vi "v2 Elevador.vi"() -> ()   [LabVIEW 2018]
panel:
  in  "Alarma":bool
  in  "NIVEL 2 2":bool
  in  "NIVEL 2 1":bool
  in  "NIVEL1 2":bool
  in  "NIVEL 1 1":bool
  in  "PLANTA BAJA 2":bool
  in  "PLANTA BAJA 1":bool
  in  "A piso 2":bool
  in  "A piso 1":bool
  in  "A planta Baja":bool
  out "Puertas Abiertas":bool
  out "Nivel actual":string
  in  "Piso 2":bool
  in  "Piso 1":bool
  in  "Planta baja":bool
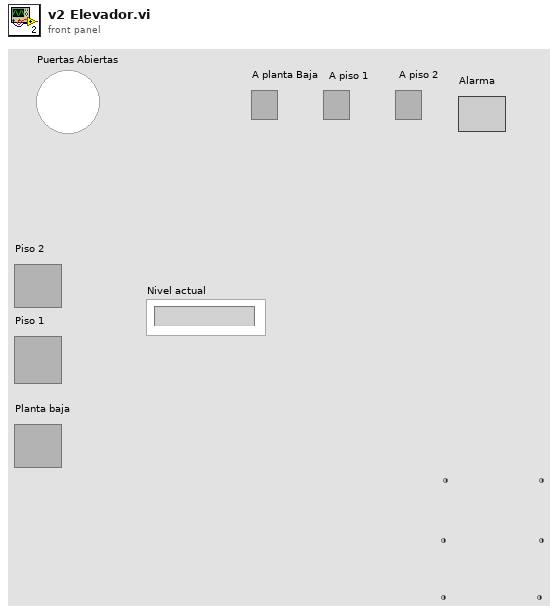
[diagram p1: front panel]
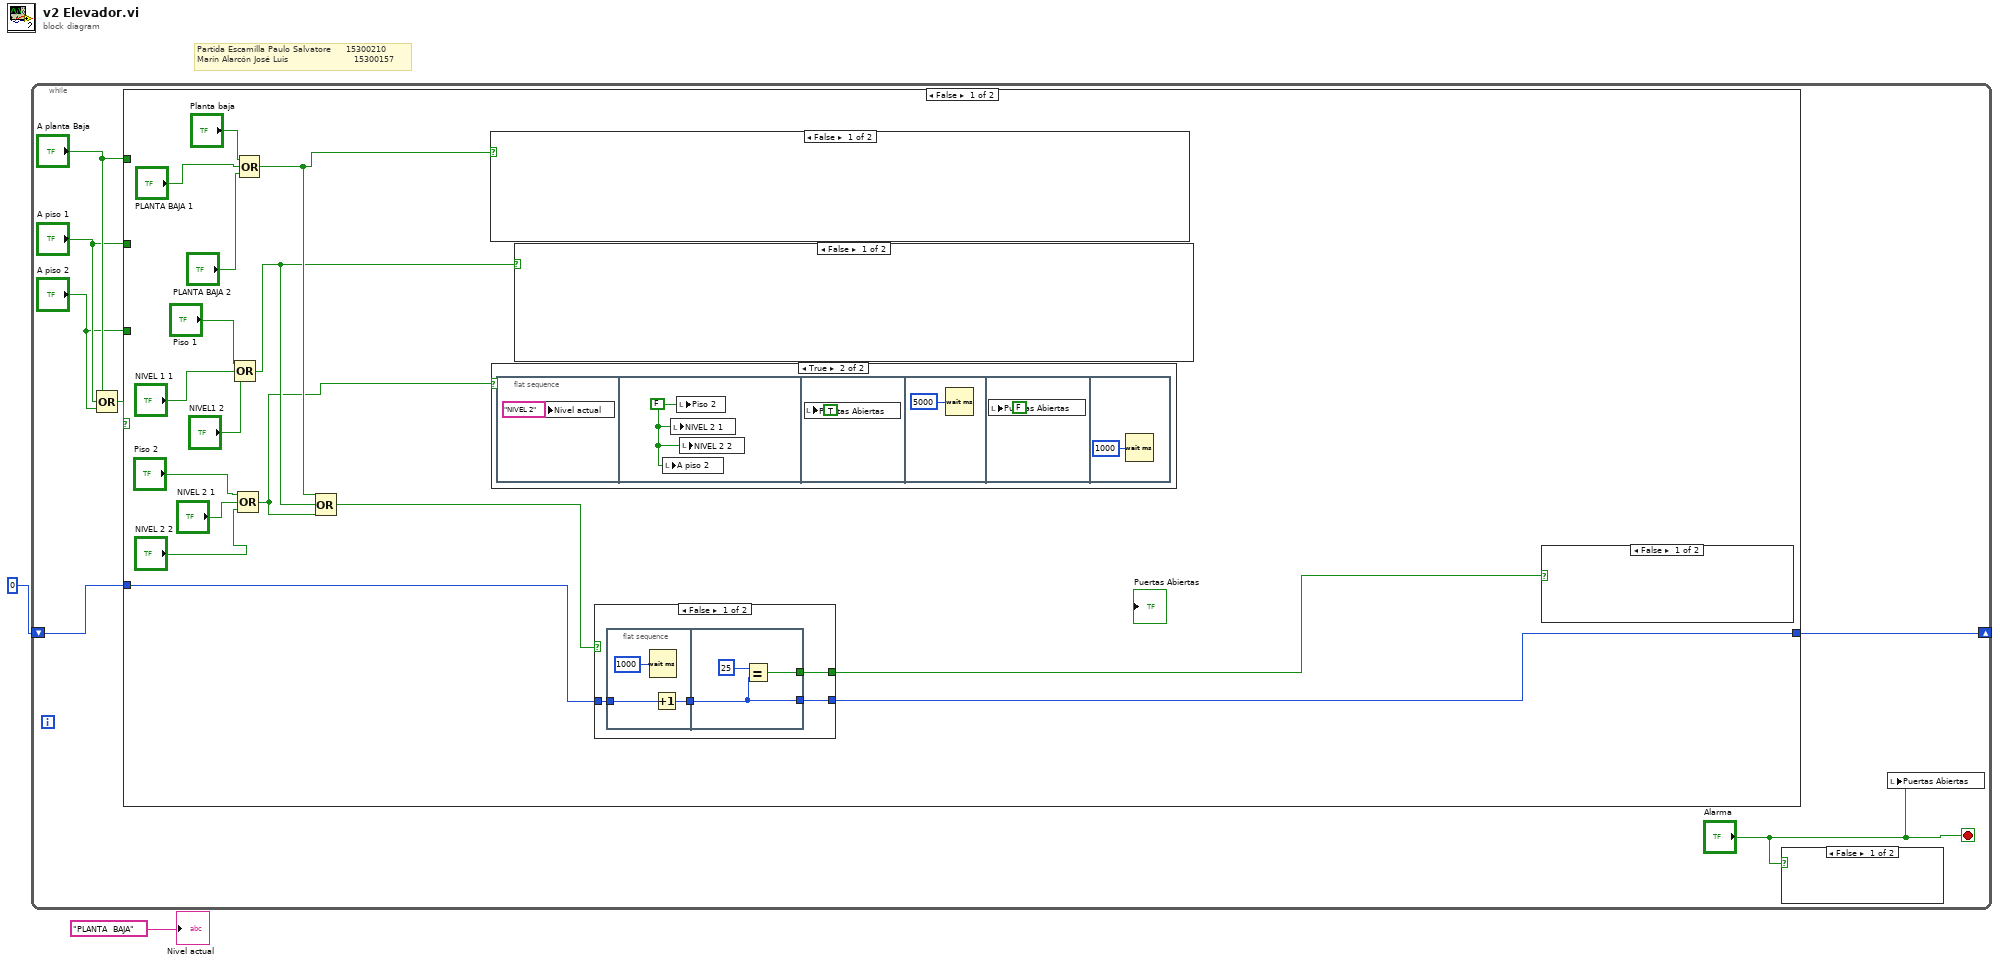
[diagram p0: block diagram]
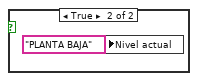
[diagram p2: hidden frame]
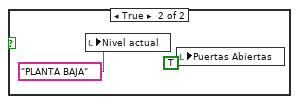
[diagram p3: hidden frame]
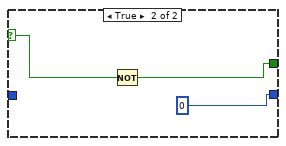
[diagram p4: hidden frame]
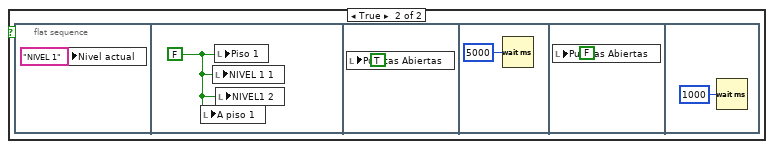
[diagram p6: hidden frame]
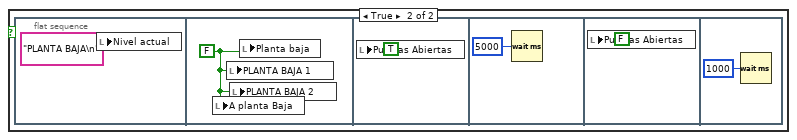
[diagram p7: hidden frame]
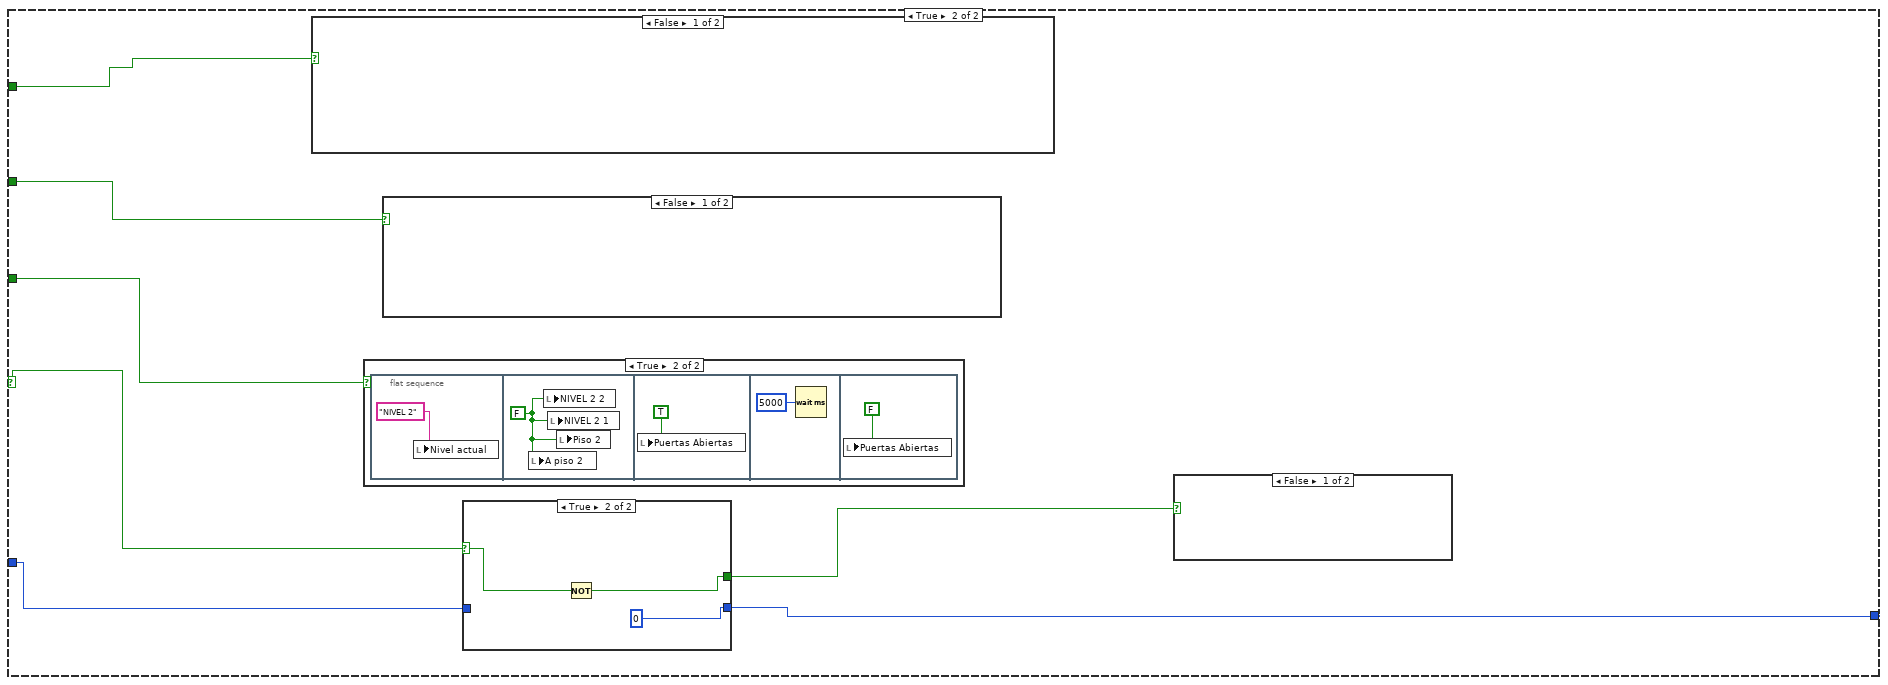
[diagram p8: hidden frame]
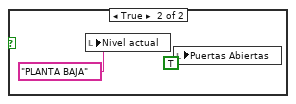
[diagram p9: hidden frame]
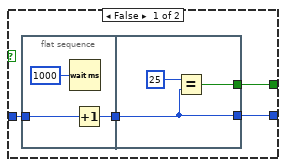
[diagram p10: hidden frame]
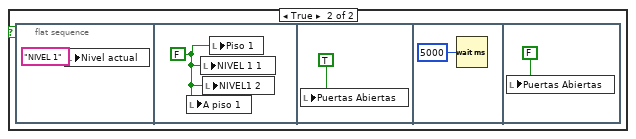
[diagram p12: hidden frame]
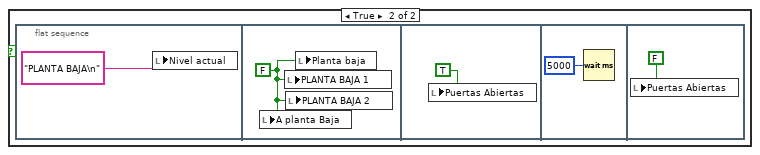
[diagram p13: hidden frame]
diagram:
  # "Partida Escamilla Paulo Salvatore     15300210\nMarín Alarcón José Luis                      15300157"
  n1 = while {
    shift-right: [w4] -> _
    shift-left: 0 -> [w5]
    stop <- "Alarma" stop-if-true
    n2 = Compound Arithmetic op=OR("A planta Baja", "A piso 1", "A piso 2") -> (w9:bool)
    n3 = case shown="False" w9 {
      selector: w9 -> [_ w62]
      tunnel: [w26 w60] -> w4
      tunnel: "A planta Baja" -> [_ w66]
      tunnel: "A piso 1" -> [_ w65]
      tunnel: "A piso 2" -> [_ w64]
      tunnel: w5 -> [w12 w63]
      frame False {
        n4 = Compound Arithmetic op=OR("Piso 1", "NIVEL 1 1", "NIVEL1 2") -> (w15:bool)
        n5 = Compound Arithmetic op=OR("Piso 2", "NIVEL 2 1", "NIVEL 2 2") -> (w14:bool)
        n6 = Compound Arithmetic op=OR("Planta baja", "PLANTA BAJA 1", "PLANTA BAJA 2") -> (w16:bool)
        n7 = Compound Arithmetic op=OR(w16, w15, w14) -> (w13:bool)
        n8 = case shown="False" w16 {
          frame False {
          }
          frame True {
            n9 = flat-sequence {
              frame #0 {
                n10 = local write "Nivel actual"("PLANTA BAJA\n" ("String")) -> ()
              }
              frame #1 {
                w55 = FALSE
                n11 = local write "A planta Baja"(w55) -> ()
                n12 = local write "PLANTA BAJA 1"(w55) -> ()
                n13 = local write "PLANTA BAJA 2"(w55) -> ()
                n14 = local write "Planta baja"(w55) -> ()
              }
              frame #2 {
                n15 = local write "Puertas Abiertas"(TRUE ("P A")) -> ()
              }
              frame #3 {
                n16 = Wait (ms)(milliseconds to wait=u32 5000) -> ()  [unwired: 1 out]
              }
              frame #4 {
                n17 = local write "Puertas Abiertas"(FALSE ("P A")) -> ()
              }
              frame #5 {
                n18 = Wait (ms)(milliseconds to wait=u32 1000) -> ()  [unwired: 1 out]
              }
            }
          }
        }
        n19 = case shown="True" w14 {
          frame False {
          }
          frame True {
            n20 = flat-sequence {
              frame #0 {
                n21 = local write "Nivel actual"("NIVEL 2" ("String")) -> ()
              }
              frame #1 {
                w43 = FALSE ("NIVEL 2")
                n22 = local write "A piso 2"(w43) -> ()
                n23 = local write "NIVEL 2 1"(w43) -> ()
                n24 = local write "Piso 2"(w43) -> ()
                n25 = local write "NIVEL 2 2"(w43) -> ()
              }
              frame #2 {
                n26 = local write "Puertas Abiertas"(TRUE ("P A")) -> ()
              }
              frame #3 {
                n27 = Wait (ms)(milliseconds to wait=u32 5000) -> ()  [unwired: 1 out]
              }
              frame #4 {
                n28 = local write "Puertas Abiertas"(FALSE ("P A")) -> ()
              }
              frame #5 {
                n29 = Wait (ms)(milliseconds to wait=u32 1000) -> ()  [unwired: 1 out]
              }
            }
          }
        }
        n30 = case shown="False" w15 {
          frame False {
          }
          frame True {
            n31 = flat-sequence {
              frame #0 {
                n32 = local write "Nivel actual"("NIVEL 1" ("String")) -> ()
              }
              frame #1 {
                w49 = FALSE
                n33 = local write "A piso 1"(w49) -> ()
                n34 = local write "NIVEL 1 1"(w49) -> ()
                n35 = local write "Piso 1"(w49) -> ()
                n36 = local write "NIVEL1 2"(w49) -> ()
              }
              frame #2 {
                n37 = local write "Puertas Abiertas"(TRUE ("P A")) -> ()
              }
              frame #3 {
                n38 = Wait (ms)(milliseconds to wait=u32 5000) -> ()  [unwired: 1 out]
              }
              frame #4 {
                n39 = local write "Puertas Abiertas"(FALSE ("P A")) -> ()
              }
              frame #5 {
                n40 = Wait (ms)(milliseconds to wait=u32 1000) -> ()  [unwired: 1 out]
              }
            }
          }
        }
        n41 = case shown="False" w13 {
          selector: w13 -> [_ w41]
          tunnel: [w32 w40] -> w11
          tunnel: [w30 0] -> w26
          tunnel: w12 -> [w29 _]
          frame False {
            n42 = flat-sequence {
              tunnel: [w34] -> w31
              tunnel: w29 -> [w33]
              tunnel: [w37] -> w32
              tunnel: w31 -> [w36]
              tunnel: [w36] -> w30
              frame #0 {
                n43 = Wait (ms)(milliseconds to wait=u32 1000) -> ()  [unwired: 1 out]
                n44 = Increment(x=w33) -> (x+1=w34:i32)
              }
              frame #1 {
                n45 = Equal?(x=25, y=w36) -> (x = y?=w37:bool)
              }
            }
          }
          frame True {
            n46 = Not(x=w41) -> (.not. x?=w40:bool)
          }
        }
        n47 = case shown="False" w11 {
          frame False {
          }
          frame True {
            n48 = local write "Nivel actual"("PLANTA BAJA" ("String")) -> ()
            n49 = local write "Puertas Abiertas"(TRUE) -> ()
          }
        }
      }
      frame True {
        n50 = case shown="False" w66 {
          frame False {
          }
          frame True {
            n51 = flat-sequence {
              frame #0 {
                n52 = local write "Nivel actual"("PLANTA BAJA\n" ("String")) -> ()
              }
              frame #1 {
                w93 = FALSE
                n53 = local write "A planta Baja"(w93) -> ()
                n54 = local write "PLANTA BAJA 1"(w93) -> ()
                n55 = local write "PLANTA BAJA 2"(w93) -> ()
                n56 = local write "Planta baja"(w93) -> ()
              }
              frame #2 {
                n57 = local write "Puertas Abiertas"(TRUE ("P A")) -> ()
              }
              frame #3 {
                n58 = Wait (ms)(milliseconds to wait=u32 5000) -> ()  [unwired: 1 out]
              }
              frame #4 {
                n59 = local write "Puertas Abiertas"(FALSE ("P A")) -> ()
              }
            }
          }
        }
        n60 = case shown="True" w64 {
          frame False {
          }
          frame True {
            n61 = flat-sequence {
              frame #0 {
                n62 = local write "Nivel actual"("NIVEL 2" ("String")) -> ()
              }
              frame #1 {
                w83 = FALSE ("NIVEL 2")
                n63 = local write "A piso 2"(w83) -> ()
                n64 = local write "NIVEL 2 2"(w83) -> ()
                n65 = local write "NIVEL 2 1"(w83) -> ()
                n66 = local write "Piso 2"(w83) -> ()
              }
              frame #2 {
                n67 = local write "Puertas Abiertas"(TRUE ("P A")) -> ()
              }
              frame #3 {
                n68 = Wait (ms)(milliseconds to wait=u32 5000) -> ()  [unwired: 1 out]
              }
              frame #4 {
                n69 = local write "Puertas Abiertas"(FALSE ("P A")) -> ()
              }
            }
          }
        }
        n70 = case shown="False" w65 {
          frame False {
          }
          frame True {
            n71 = flat-sequence {
              frame #0 {
                n72 = local write "Nivel actual"("NIVEL 1" ("String")) -> ()
              }
              frame #1 {
                w88 = FALSE
                n73 = local write "A piso 1"(w88) -> ()
                n74 = local write "NIVEL 1 1"(w88) -> ()
                n75 = local write "NIVEL1 2"(w88) -> ()
                n76 = local write "Piso 1"(w88) -> ()
              }
              frame #2 {
                n77 = local write "Puertas Abiertas"(TRUE ("P A")) -> ()
              }
              frame #3 {
                n78 = Wait (ms)(milliseconds to wait=u32 5000) -> ()  [unwired: 1 out]
              }
              frame #4 {
                n79 = local write "Puertas Abiertas"(FALSE ("P A")) -> ()
              }
            }
          }
        }
        n80 = case shown="True" w62 {
          selector: w62 -> [_ w81]
          tunnel: [w72 w80] -> w61
          tunnel: [w70 0] -> w60
          tunnel: w63 -> [w69 _]
          frame False {
            n81 = flat-sequence {
              tunnel: [w74] -> w71
              tunnel: w69 -> [w73]
              tunnel: [w77] -> w72
              tunnel: w71 -> [w76]
              tunnel: [w76] -> w70
              frame #0 {
                n82 = Wait (ms)(milliseconds to wait=u32 1000) -> ()  [unwired: 1 out]
                n83 = Increment(x=w73) -> (x+1=w74:i32)
              }
              frame #1 {
                n84 = Equal?(x=25, y=w76) -> (x = y?=w77:bool)
              }
            }
          }
          frame True {
            n85 = Not(x=w81) -> (.not. x?=w80:bool)
          }
        }
        n86 = case shown="False" w61 {
          frame False {
          }
          frame True {
            n87 = local write "Nivel actual"("PLANTA BAJA" ("String")) -> ()
            n88 = local write "Puertas Abiertas"(TRUE) -> ()
          }
        }
      }
    }
    n89 = case shown="False" "Alarma" {
      frame False {
      }
      frame True {
        n90 = local write "Nivel actual"("PLANTA BAJA" ("String")) -> ()
      }
    }
    n91 = local write "Puertas Abiertas"("Alarma") -> ()
  }
  "Nivel actual" <- "PLANTA  BAJA" ("String")
